vi "TagGetResponse_Parse.vi"(8 "error in (no error)":errorcluster, 11 "Message":T6) -> (0 "error out":errorcluster, 1 "Body":T1, 2 "Header":T5, 3 "TagGetResponse":T4)   [LabVIEW 2017]
uses:
  <vilib>/addons/InsightCM/MessageBus/Base/controls/Message.ctl
  <vilib>/addons/InsightCM/MessageBus/Base/controls/MessageHeader.ctl
  <vilib>/addons/InsightCM/MessageBus/Base/controls/KeyValuePair.ctl
  <vilib>/addons/InsightCM/MessageBus/MessageLibrary/Tag/controls/TagGetResponse.ctl
  <vilib>/addons/InsightCM/MessageBus/MessageLibrary/Tag/controls/TagGetResponseBody.ctl
  <vilib>/addons/InsightCM/MessageBus/Base/controls/Tag.ctl
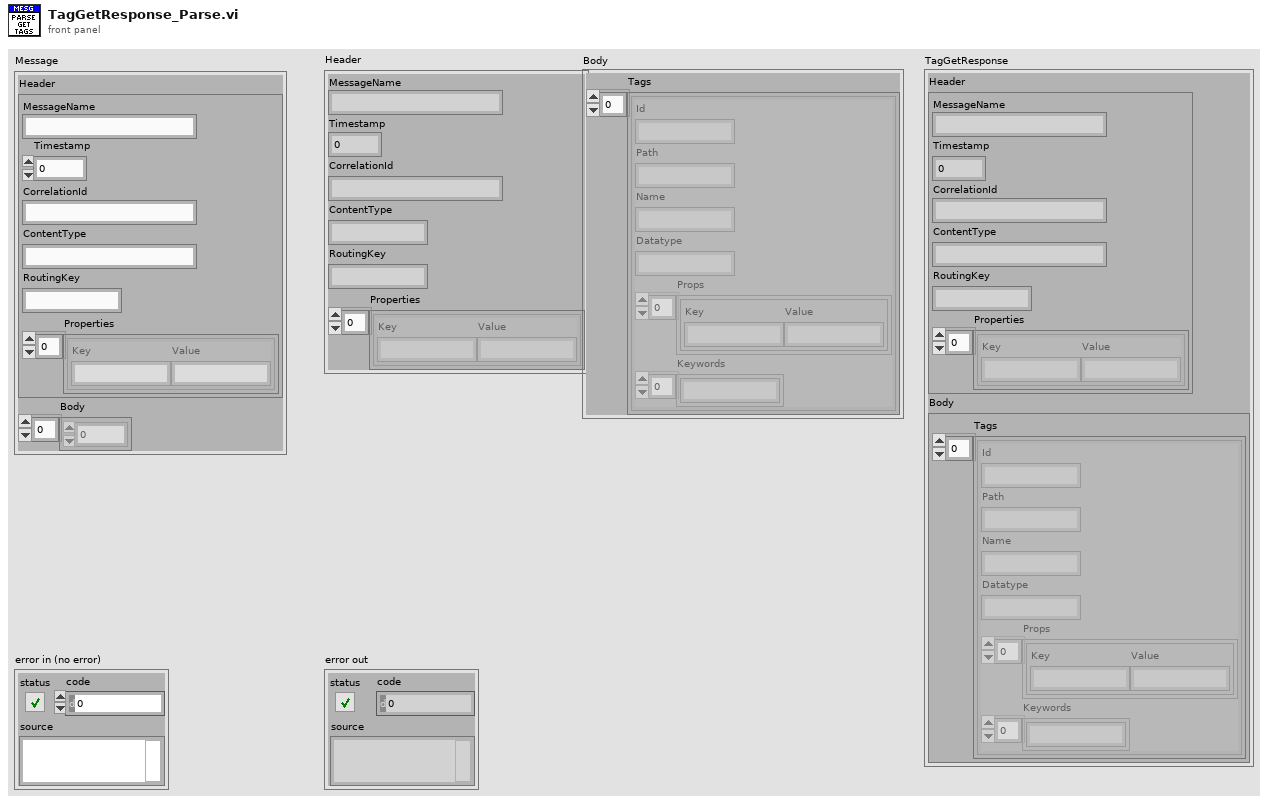
[diagram p1: front panel]
types:
  T1 = typedef "TagGetResponseBody.ctl" = cluster{"Tags":T2[]}
  T2 = typedef "Tag.ctl" = cluster{"Id":string, "Path":string, "Name":string, "Datatype":string, "Props":T3[], "Keywords":string[]}
  T3 = typedef "KeyValuePair.ctl" = cluster{"Key":string, "Value":string}
  T4 = typedef "TagGetResponse.ctl" = cluster{"Header":T5, "Body":T1}
  T5 = typedef "MessageHeader.ctl" = cluster{"MessageName":string, "Timestamp":i64, "CorrelationId":string, "ContentType":string, "RoutingKey":string, "Properties":T3[]}
  T6 = typedef "Message.ctl" = cluster{"Header":T5, "Body":u8[]}
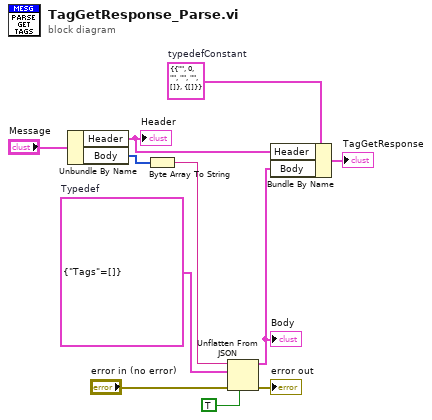
[diagram p0: block diagram]
diagram:
  w3 = T4 {"Header"={"MessageName"="", "Timestamp"=0, "CorrelationId"="", "ContentType"="", "RoutingKey"="", "Properties"=[]}, "Body"={"Tags"=[]}}  # typedefConstant
  w7 = T1 {"Tags"=[]}  # Typedef
  n1 = Unbundle By Name("Message") -> ("Header"=w9:T5, "Body"=w1:u8[])
  "Header" <- w9
  n2 = Byte Array To String(unsigned byte array=w1) -> (string=w6:string)
  n3 = Unflatten From JSON(JSON string=w6, type and defaults=w7, default null elements? (F)=TRUE, error in (no error)="error in (no error)") -> (value=w5:T1, error out=→"error out":errorcluster)  [unwired: 3 in]
  "Body" <- w5
  n4 = Bundle By Name(cluster=w3, "Header"=w9, "Body"=w5) -> (→"TagGetResponse":T4)
